vi "Add time.vi"(8 "error in (no error)":errorcluster, 10 "Numeric Control":u32, 11 "Timer in":refnum<class "Timer.lvclass">) -> (0 "error out":errorcluster, 3 "Timer out":refnum<class "Timer.lvclass">)   [LabVIEW 2018, in "Timer.lvclass"]
uses:
  Timer.lvclass
  Timer.lvclass/Timer.ctl
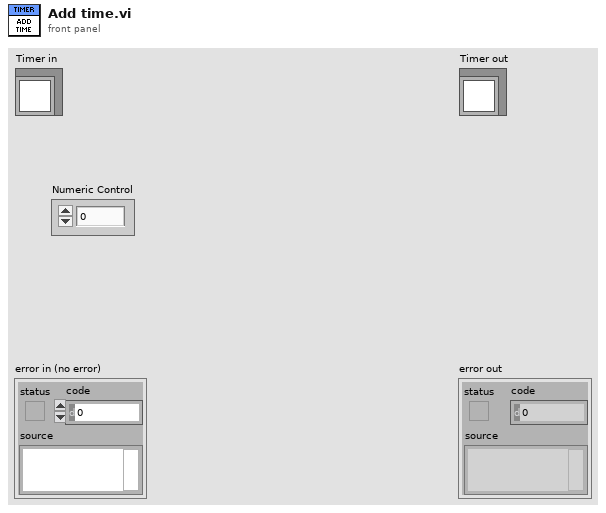
[diagram p1: front panel]
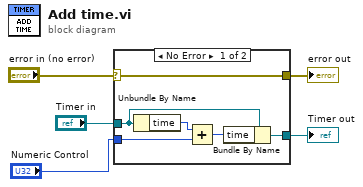
[diagram p0: block diagram]
diagram:
  n1 = case shown="No Error" "error in (no error)" {
    selector: "error in (no error)" -> [w11 w13]
    tunnel: [w11 w13] -> w4
    tunnel: [w10 w12] -> w2
    tunnel: "Timer in" -> [w6 w12]
    tunnel: "Numeric Control" -> [w8 _]
    frame No Error {
      n2 = Unbundle By Name(w6) -> ("time"=w9:u32)
      n3 = Add(x=w9, y=w8) -> (x+y=w7:u32)
      n4 = Bundle By Name(cluster=w6, "time"=w7) -> (w10:refnum<class "Timer.lvclass">)
    }
    frame Error {
    }
  }
  "error out" <- w4
  "Timer out" <- w2
